vi "Idle Reference Image Window.vi"() -> ()   [LabVIEW 2017]
uses:
  Typedefs/Channel Selector.ctl
  Queue/Message Queue/Typedefs/Message Cluster.ctl
  SubVIs/Typedefs/Live window-ctrl refs.ctl
  Typedefs/Image display ref.ctl
  Typedefs/Save-Load enum.ctl
  <vilib>/Utility/miscctls.llb/LVPointTypeDef.ctl
  Typedefs/Read Write Enum.ctl
  Typedefs/Channel control synergistic behaviour enum.ctl
  Typedefs/Top level VI states.ctl
  Globals/gl_Windows Ctrl refs.vi
  Global Variables/General Globals.vi
  Global Variables/gl_UI Ctrl Refs.vi
panel:
  in  "UI queue ref control":refnum<queue>
  in  "Stop":bool
  in  "Show REF Image Right":bool caption="Show REF Image"
  in  "Show REF Image Left":bool caption="Show REF Image"
  in  "Base Path":path
  out "Frame rate (Hz)":dbl format="Acquisition frame rate: %.1f fps"
  in  "Sim multiplier":dbl(knob) scale=0.1..10.0
  out "Loop":i32
  out "Reset buffer":bool
  out "Refresh rate (Hz)":i32 format="Graph refresh rate: %.0f fps"
  in  "Right image intensity":cluster{i16, i16}(slide)={0, 804} scale=0.0..4095.0
  in  "Right Image Palette":enum16{"Gray", "Red", "Green"}(ring) caption="Palette"
  in  "Right Channel":T1=enum."Green Channel"
  in  "Left image intensity":cluster{i16, i16}(slide)={0, 871} scale=0.0..4095.0
  in  "Left Image Palette":enum16{"Gray", "Red", "Green"}(ring) caption="Palette"
  in  "Left Channel":T1
  in  "Y-scaling sensitivity":i32(slide)=32 scale=100.0..1.0
  in  "Sim":bool
  in  "AutoY once":bool
  in  "Selected Waveform":enum16{"Left graph", "Right graph"}(ring) caption="Displayed data"
  in  "Adaptive scaling is on":bool
  out "multiple tone information":T2(array[cluster])=[{"detected frequency"=59.40457132494078, "detected amplitude"=677.5224683183739, "detected phase (deg)"=-6.85916777032908}, {"detected frequency"=10023.302847711435, "detected amplitude"=302.0949374874943, "detected phase (deg)"=265.4481634375171}, {"detected frequency"=20019.602268100927, "detected amplitude"=136.99007273675608, "detected phase (deg)"=123.98051462950585}, {"detected frequency"=30006.01918128676, "detected amplitude"=20.477000538882503, "detected phase (deg)"=-16.173557072223005}] {"detected phase (deg)" format="%_6g"; "detected amplitude" format="%_6p"; "detected frequency" format="%_6p"}
  out "Right Image":T3(plugin-control)
  in  "Snapshot":bool
  out "Left Image":T3(plugin-control)
  out "Data graph":waveform(dbl)(graph)
  # "DO NOT DELETE THIS CONTROL. IT IS REFERENCED."
  # "Low                                   High"
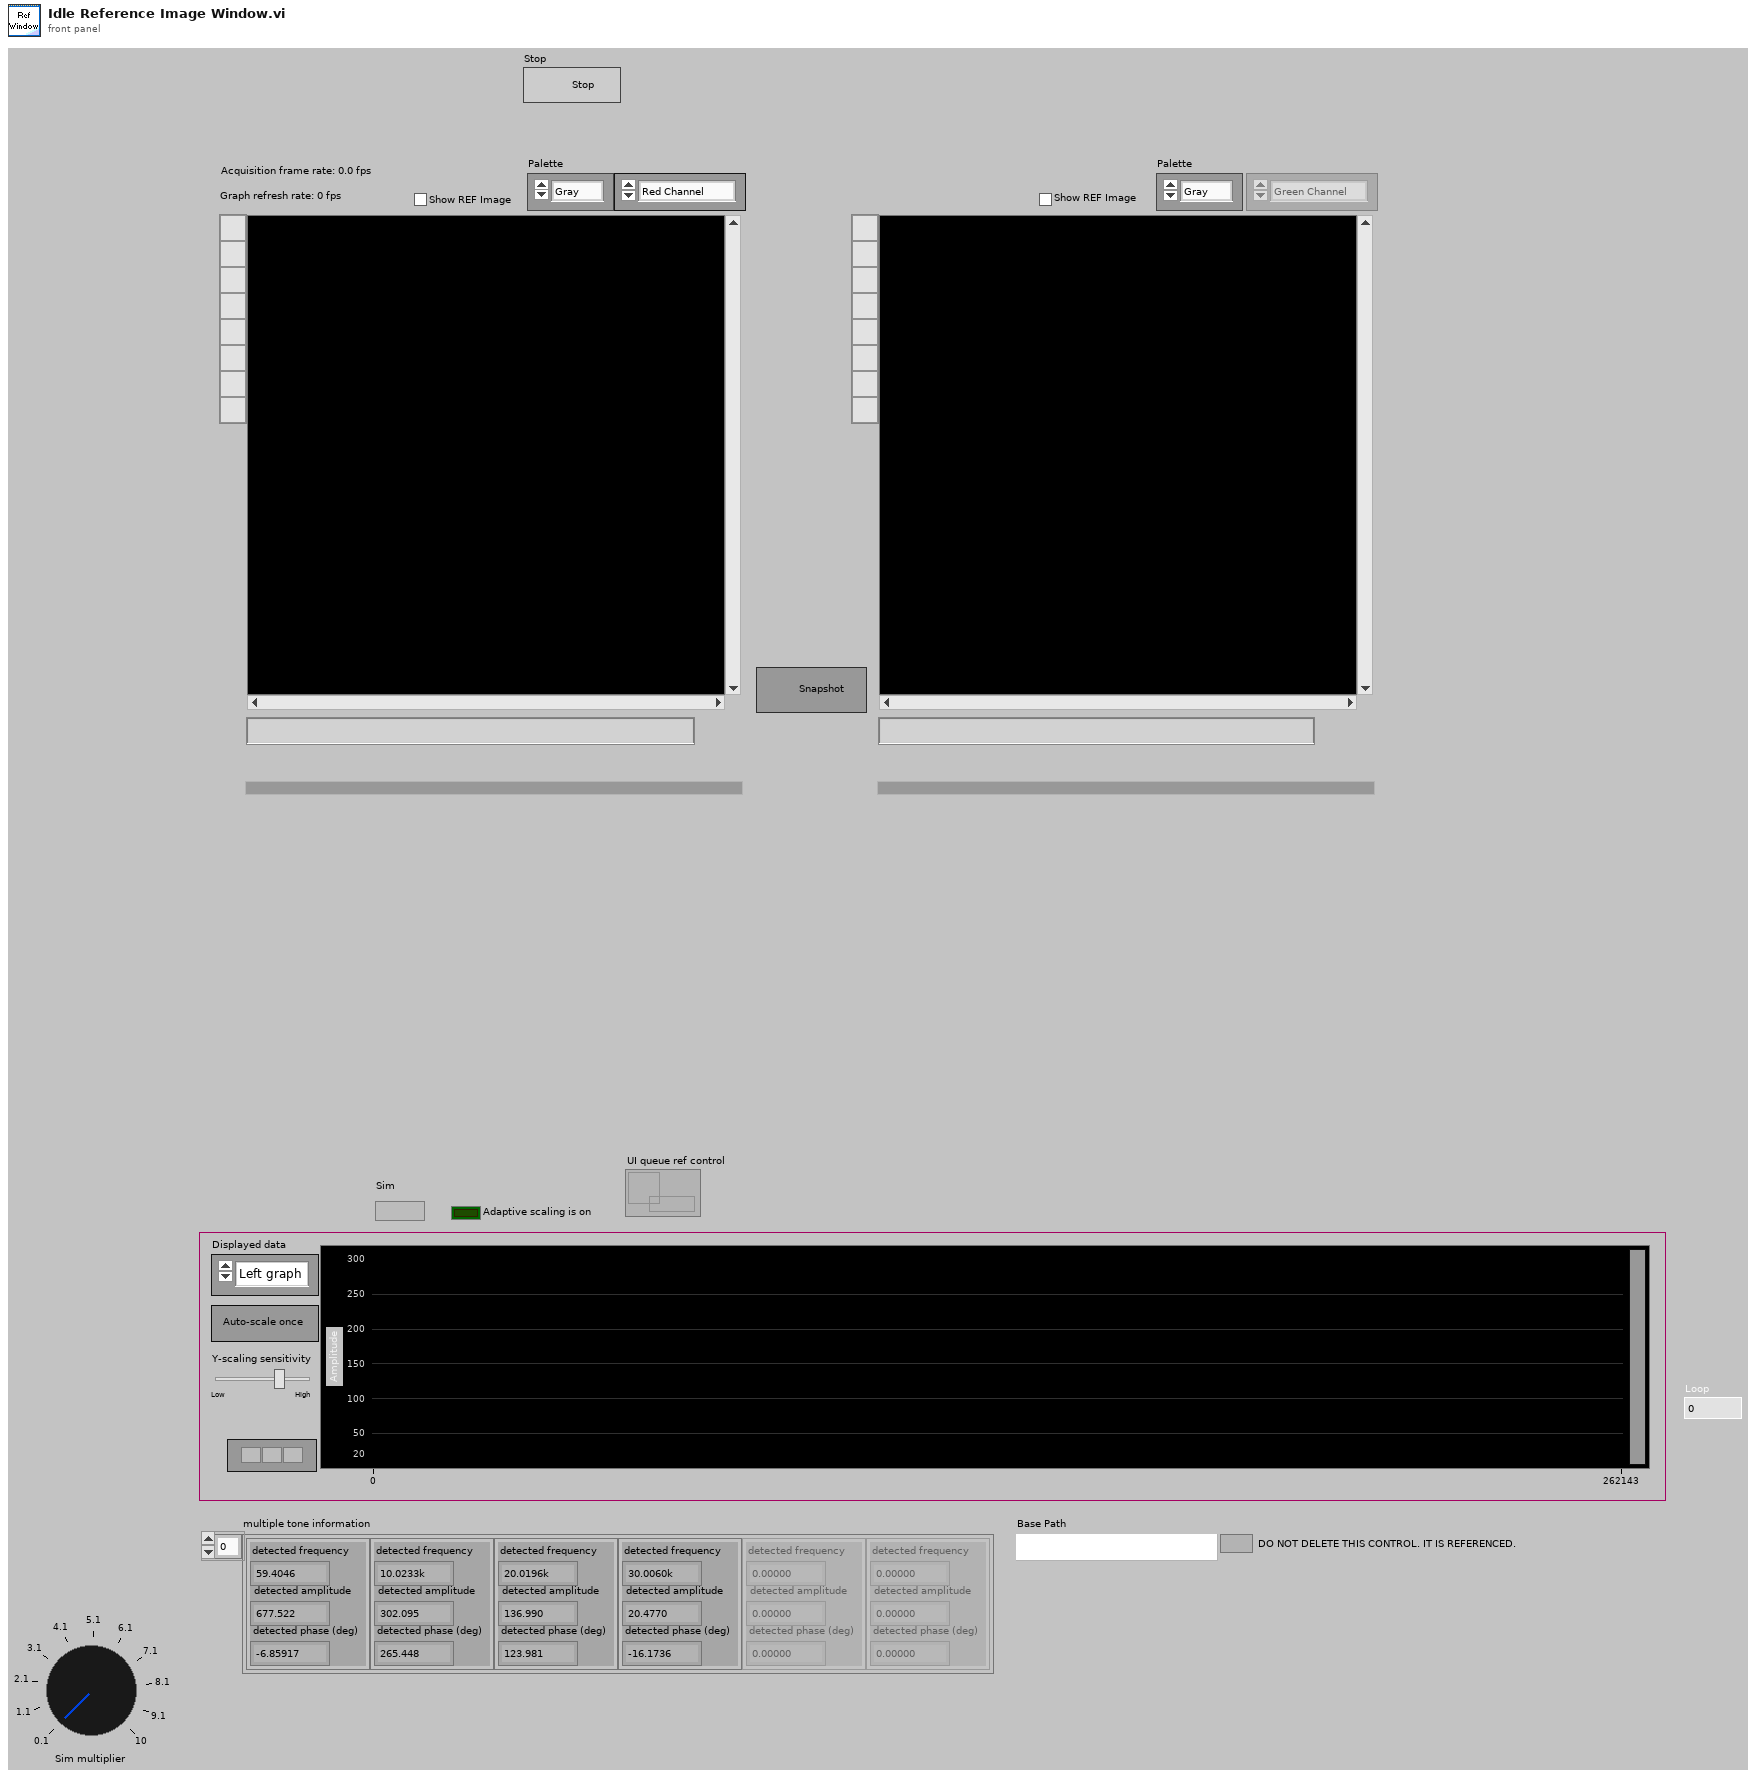
[diagram p1: front panel]
types:
  T1 = typedef "Channel Selector.ctl" = enum16{"Red Channel", "Green Channel", "Blended"}
  T2 = cluster{"detected frequency":dbl, "detected amplitude":dbl, "detected phase (deg)":dbl}[]
  T3 = typedef "IMAQ Image.ctl" = refnum<image>
  T4 = typedef "Live window-ctrl refs.ctl" = cluster{"This VI":refnum<vi>, "Pane":refnum<vi>, "Show REF Image Left":refnum<vi>, "Show REF Image Right":refnum<vi>, "Snapshot":refnum<vi>, "Left Image Palette":refnum<vi>, "Right Image Palette":refnum<vi>, "Left Channel":refnum<vi>, "Right Channel":refnum<vi>, "Left image intensity":refnum<vi>, "Right image intensity":refnum<vi>, "Left Image Display":T5, "Right Image Display":T5, "Refresh rate ind (Hz)":refnum<vi>, "Acq rate ind (Hz)":refnum<vi>, "Stop (ind)":refnum<vi>}
  T5 = typedef "Image display ref.ctl" = refnum<vi>
  T6 = typedef "Save-Load enum.ctl" = enum16{"Save to file", "Load from file", "Compare from file"}
  T7 = typedef "Read Write Enum.ctl" = enum16{"Read", "Write"}
  T8 = cluster{"Conversion Method":u32, "Minimum Value":i32, "Maximum Value":i32, "Number Of Shifts":i32}
  T9 = typedef "LVPointTypeDef.ctl" = cluster{"Horizontal":i16, "Vertical":i16}
  T10 = typedef "UI ctrl refs cluster.ctl" = cluster{"Top level VI path":path, "Top level VI ref":refnum<vi>, "User menu ref":refnum<k9>, "Sub Panel control":refnum<vi>, "Imaging Param Tab":refnum<vi>, "Occurrence-Start drivers":refnum<k4>, "Occurrence-Speed logging initialised":refnum<k4>, "Occurrence-XYZ stage initialised":refnum<k4>, "Exit button":refnum<vi>, "Status ind":refnum<vi>, "Set as origin":refnum<vi>, "Speed Logging":refnum<vi>, "Time Lapse":refnum<vi>, "Live Imaging":refnum<vi>, "AOL Z Stack":refnum<vi>, "Motor Z Stack":refnum<vi>, "Funct Acq button":refnum<vi>, "Hard Shutter":refnum<vi>, "Virtual Shutter":refnum<vi>, "Laser Power":refnum<vi>, "AOL Mode":refnum<vi>, "Frame Size":refnum<vi>, "Field of View":refnum<vi>, "Dwell Time":refnum<vi>, "Zoom":refnum<vi>, "AOL Z":refnum<vi>, "Objective":refnum<vi>, "Axis":refnum<vi>, "Paths & Names":refnum<vi>, "Experiment folder path (ind.)":refnum<vi>, "Last State (Ind.)":refnum<vi>, "Averages":refnum<vi>, "Angle (degrees)":refnum<vi>, "X centre":refnum<vi>, "Y centre":refnum<vi>, "Plane Mode":refnum<vi>, "# Planes":refnum<vi>, "Z Start":refnum<vi>, "Z Stop":refnum<vi>, "Z Step":refnum<vi>, "PMT 1":refnum<vi>, "PMT 2":refnum<vi>, "Stage XYZ Position":refnum<vi>, "Pockels@Z Start":refnum<vi>, "Pockels@Z Stop":refnum<vi>, "Obtain Z Start":refnum<vi>, "Obtain Z Stop":refnum<vi>, "Live stim.trig.period":refnum<vi>, "Live stim.trig.enable":refnum<vi>, "Movement Correction":refnum<vi>, "Load Reference Image":refnum<vi>, "XY Stage Move":refnum<vi>, "MovCor Cluster":refnum<vi>, "RefDAQParam":refnum<vi>, "Funct. Acq. Pockels Modulation":refnum<vi>, "Ref Laser Power":refnum<vi>, "Enable Video Recording":refnum<vi>, "Video Record-Live Imaging":refnum<vi>, "Video Record-Funct acq":refnum<vi>, "Reference Source":refnum<vi>, "AOL Z-stack Chirps Ready (ind)":refnum<vi>, "Target time between mov.cor. ref triggers (ms)":refnum<vi>, "Funct. Acq. Ref frame save":refnum<vi>, "Tracking button":refnum<vi>, "Show ref plots window":refnum<vi>, "Center freq ind (nm)":refnum<vi>, "Pickup mode (ind)":refnum<vi>, "Logging queue (ind)":refnum<vi>, "Back aperture power (ind.)":refnum<vi>, "Power after objective (ind.)":refnum<vi>, "Switch user":refnum<vi>, "Ls1 Conn. Status":refnum<vi>, "Ls1Tuning Status":refnum<vi>, "Ls1 Faults":refnum<vi>, "Ls1 Connection":refnum<vi>, "Ls1 Mode":refnum<vi>, "Ls1 POWER [mW]":refnum<vi>, "Ls1Shutter":refnum<vi>, "Ls1 Wavelength":refnum<vi>, "Ls1 Note":refnum<vi>, "Ls1 Confirm Wav":refnum<vi>, "Ls1 PreChrp Prism1":refnum<vi>, "Ls1 PreChrp Prism2":refnum<vi>, "Ls1 wav top Ind":refnum<vi>, "Ls1 power top Ind":refnum<vi>, "Ls1 Pump peak Hold":refnum<vi>, "Ls1 Status Ind":refnum<vi>, "Ls1 wav cancel":refnum<vi>, "Experiment Type":refnum<vi>, "Biology Information":refnum<vi>}
  T11 = typedef "Live graph data queue ref.ctl" = refnum<queue>
  T12 = typedef "Channel control synergistic behaviour enum.ctl" = enum16{"Left disabled-Right enabled", "Left enabled-Right disabled", "Both enabled"}
  T13 = cluster{"Caption-Right button":string, "Caption-Left button":string, "Message to display":string, "Delay before close":u32, "Window Colour":u32, "Cancel button disabled?":enum8{"Enabled", "Disabled", "Disabled and Grayed Out"}}
  T14 = typedef "Top level VI states.ctl" = enum16{"None", "Initialise UI", "<STACK PROTOCOL STATES>", "AOL Zstack-START", "AOL Zstack-STOP", "Motor Zstack-START", "Motor Zstack-STOP", "<ACQUISITION PROTOCOL STATES> ", "Functional Acquisition-START", "Functional Acquisition-STOP", "Single Plane Acquisition-START", "Single Plane Acquisition-STOP", "Volume Acquisition-START", "Volume Acquisition-STOP", "<LIVE IMAGING PROTOCOL STATES>", "Live Imaging-START", "Live Imaging-STOP", "Live Plane Imaging-START", "Live Plane Imaging-STOP", "Live Volume Imaging-START", "Live Volume Imaging-STOP", "<MOVEMENT CORRECTION PROTOCOL STATES>", "EXIT"}
  T15 = typedef "Live imaging queue element.ctl" = cluster{"Red channel":T3, "Green channel":T3, "Ref Red channel":T3, "Ref Green channel":T3, "Mov cor":bool}
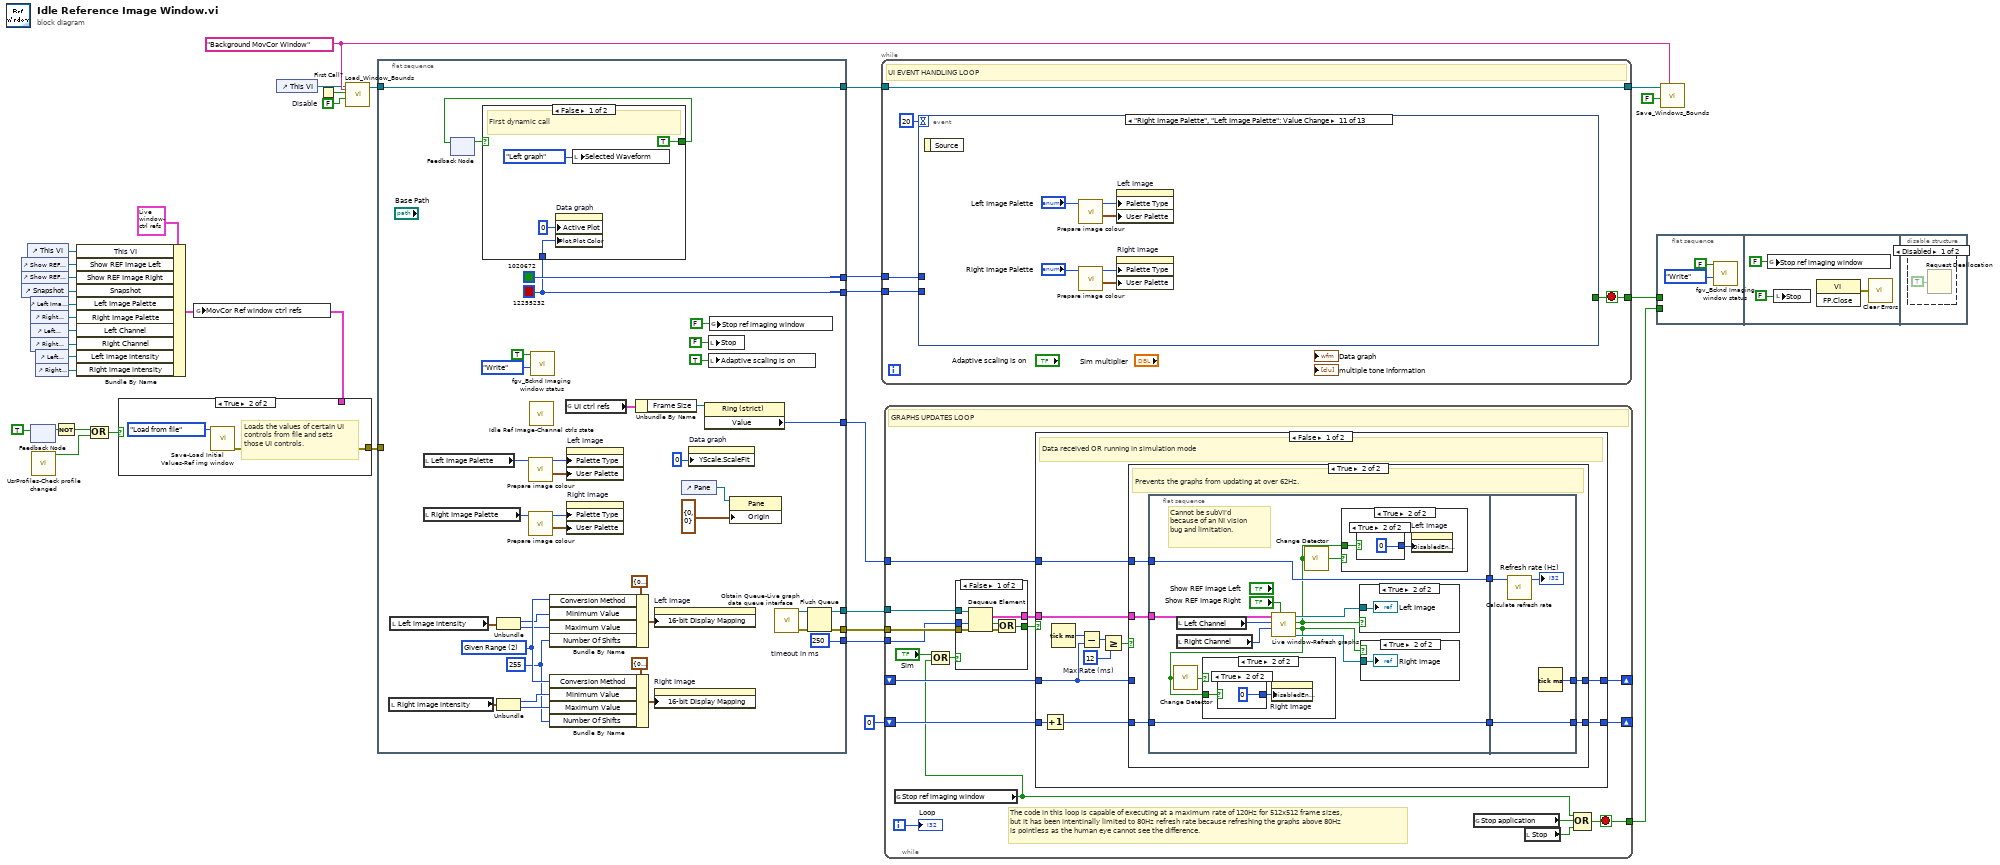
[diagram p0: block diagram]
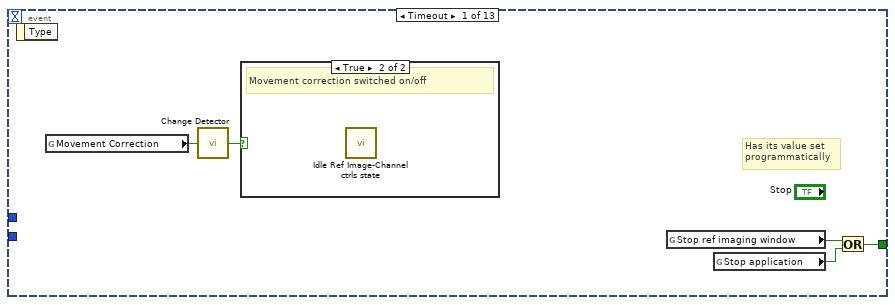
[diagram p5: hidden frame]
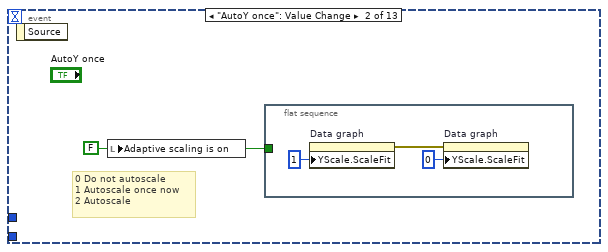
[diagram p7: hidden frame]
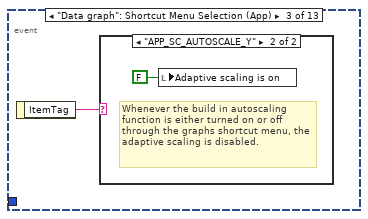
[diagram p8: hidden frame]
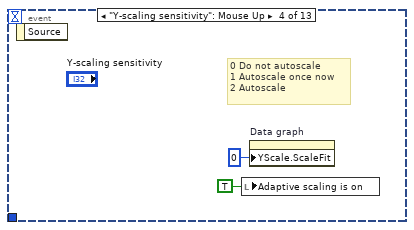
[diagram p10: hidden frame]
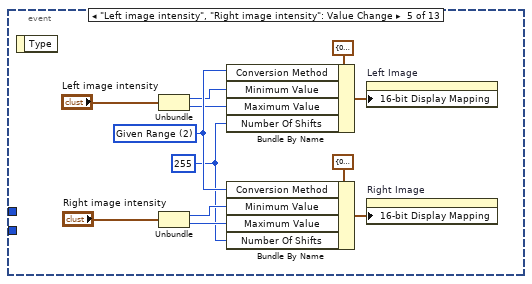
[diagram p11: hidden frame]
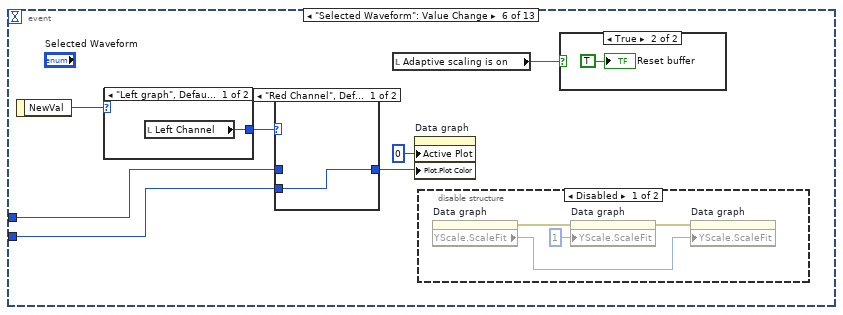
[diagram p12: hidden frame]
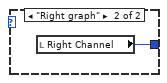
[diagram p16: hidden frame]
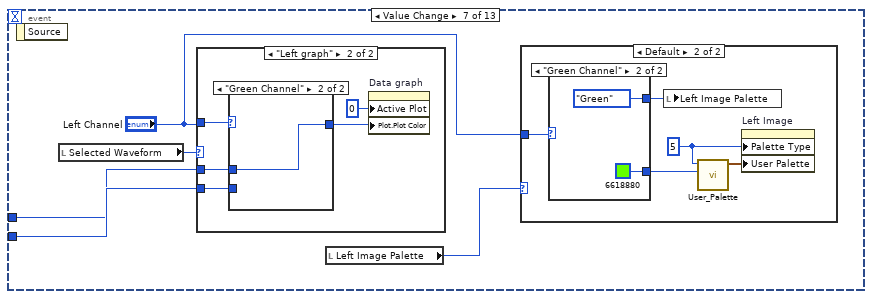
[diagram p17: hidden frame]
diagram:
  w31 = FALSE  # Disable
  w30 = "Background MovCor Window" ("Window Name (i.e. Key)")
  n1 = control-ref of="Show REF Image Left"() -> (w15:refnum<vi>)
  n2 = control-ref of="Show REF Image Right"() -> (w16:refnum<vi>)
  n3 = control-ref of="Snapshot"() -> (w17:refnum<vi>)
  n4 = control-ref of="This VI"() -> (w14:refnum<vi>)
  n5 = control-ref of="Left Image Palette"() -> (w11:refnum<vi>)
  n6 = control-ref of="Right Image Palette"() -> (w10:refnum<vi>)
  n7 = control-ref of="Left Channel"() -> (w9:refnum<vi>)
  n8 = control-ref of="Right Channel"() -> (w8:refnum<vi>)
  n9 = feedback #1() -> (w5:bool)  [unwired: 1 in]
  n10 = feedback-in #1(TRUE) -> ()
  n11 = call "UsrProfiles-Check profile changed.vi"() -> ("Profile changed"=w1:bool)  [unwired: 10 in, 1 out]
  n12 = control-ref of="Left image intensity"() -> (w7:refnum<vi>)
  n13 = control-ref of="Right image intensity"() -> (w6:refnum<vi>)
  n14 = Not(x=w5) -> (.not. x?=w3:bool)
  n15 = Bundle By Name(cluster=T4 {"This VI"=refnum, "Pane"=refnum, "Show REF Image Left"=refnum, "Show REF Image Right"=refnum, "Snapshot"=refnum, "Left Image Palette"=refnum, "Right Image Palette"=refnum, "Left Channel"=refnum, "Right Channel"=refnum, "Left image intensity"=refnum, "Right image intensity"=refnum, "Left Image Display"=refnum, "Right Image Display"=refnum, "Refresh rate ind (Hz)"=refnum, "Acq rate ind (Hz)"=refnum, "Stop (ind)"=refnum} ("Live imaging window ctrl refs"), "This VI"=w14, "Show REF Image Left"=w15, "Show REF Image Right"=w16, "Snapshot"=w17, "Left Image Palette"=w11, "Right Image Palette"=w10, "Left Channel"=w9, "Right Channel"=w8, "Left image intensity"=w7, "Right image intensity"=w6) -> (w12:T4)
  n16 = Compound Arithmetic op=OR(w3, w1) -> (w2:bool)
  n17 = case shown="True" w2 {
    tunnel: [_ w36] -> w18
    tunnel: w12 -> [_ _]
    frame False {
    }
    frame True {
      # "Loads the values of certain UI controls from file and sets those UI controls."
      n18 = call "Save-Load Initial Values-Ref img window.vi"("Function"=Save-Load_enum."Load from file") -> ("error out"=w36:errorcluster)  [unwired: 10 in]
    }
  }
  n19 = global write "gl_Windows Ctrl refs.vi" "MovCor Ref window ctrl refs"(w12) -> ()
  n20 = control-ref of="This VI"() -> (w24:refnum<vi>)
  n21 = First Call?() -> (First Call?: T/F=w32:bool)
  n22 = call "Load_Window_Bounds.vi"("Window Name (i.e. Key)"=w30, "Disable"=w31, "First Call"=w32, "Window VI's Ref"=w24) -> ("reference out"=w19:refnum<vi>)  [unwired: 4 in, 3 out]
  n23 = flat-sequence {
    tunnel: [u32 1020672 ("Green")] -> w35
    tunnel: [w75] -> w34
    tunnel: [w72] -> w33
    tunnel: w19 -> [w44]
    tunnel: [w44] -> w23
    tunnel: [w41] -> w22
    tunnel: [w40] -> w21
    tunnel: [w42] -> w20
    tunnel: w18 -> [_]
    frame #0 {
      w42 = 250  # timeout in ms
      w57 = 255 ("Number Of Shifts")
      w65 = u32 2 items=["Full Dynamic", "Downshift", "Given Range", "90% Dynamic", "Given Percent Range"] ("16-bit Display Mapping:Conversion Method")
      w75 = u32 12255232 ("Red")
      n24 = local read "Right image intensity"() -> (w67:cluster{i16, i16})
      n25 = local read "Left image intensity"() -> (w66:cluster{i16, i16})
      n26 = local read "Left Image Palette"() -> (w49:enum16{"Gray", "Red", "Green"})
      n27 = local read "Right Image Palette"() -> (w48:enum16{"Gray", "Red", "Green"})
      n28 = feedback #2() -> (w74:bool)  [unwired: 1 in]
      n29 = case shown="False" w74 {
        selector: w74 -> [_ w81]
        tunnel: w75 -> [w78 _]
        tunnel: [TRUE w81] -> w73
        frame False {
          # "First dynamic call"
          n30 = property on="Data graph" class="MixedGraph (strict)"("Active Plot"=u32 0, "Plot.Plot Color"=w78) -> ()  [unwired: 2 in, 2 out]
          n31 = local write "Selected Waveform"(enum16{"Left graph", "Right graph"}."Left graph" ("Selected Waveform")) -> ()
        }
        frame True {
          # "Consecutive calls"
        }
      }
      n32 = feedback-in #2(w73) -> ()
      n33 = Unbundle(w66) -> (w61:i16, w62:i16)
      n34 = Unbundle(w67) -> (w64:i16, w63:i16)
      n35 = call "Prepare image colour.vi"("Left Image Palette"=w49) -> ("Color Palette"=w52:cluster{"Red":u8, "Green":u8, "Blue":u8}[], "Palette Type"=w50:u32)  [unwired: 8 in, 1 out]
      n36 = call "Prepare image colour.vi"("Left Image Palette"=w48) -> ("Color Palette"=w53:cluster{"Red":u8, "Green":u8, "Blue":u8}[], "Palette Type"=w51:u32)  [unwired: 8 in, 1 out]
      n37 = call "Idle Ref Image-Channel ctrls state.vi"() -> ()  [unwired: 12 in]
      n38 = call "fgv_Bcknd Imaging window status.vi"("Function"=Read_Write_Enum."Write", "Background MovCor window is open"=TRUE) -> ()  [unwired: 8 in, 2 out]
      n39 = Bundle By Name(cluster=T8 {"Conversion Method"=0, "Minimum Value"=0, "Maximum Value"=0, "Number Of Shifts"=0} ("16-bit Display Mapping:All Elements"), "Conversion Method"=w65, "Minimum Value"=w61, "Maximum Value"=w62, "Number Of Shifts"=w57) -> (w59:T8)
      n40 = Bundle By Name(cluster=T8 {"Conversion Method"=0, "Minimum Value"=0, "Maximum Value"=0, "Number Of Shifts"=0} ("16-bit Display Mapping:All Elements"), "Conversion Method"=w65, "Minimum Value"=w64, "Maximum Value"=w63, "Number Of Shifts"=w57) -> (w58:T8)
      n41 = global read "gl_UI Ctrl Refs.vi" "UI ctrl refs"() -> (w54:T10)
      n42 = property on="Left Image" class="ImageControl"("Palette Type"=w50, "User Palette"=w52) -> ()  [unwired: 2 in, 2 out]
      n43 = property on="Right Image" class="ImageControl"("Palette Type"=w51, "User Palette"=w53) -> ()  [unwired: 2 in, 2 out]
      n44 = Unbundle By Name(w54) -> ("Frame Size"=w55:refnum<vi>)
      n45 = property on="Left Image" class="ImageControl"("16-bit Display Mapping"=w59) -> ()  [unwired: 2 in, 2 out]
      n46 = property on="Right Image" class="ImageControl"("16-bit Display Mapping"=w58) -> ()  [unwired: 2 in, 2 out]
      n47 = control-ref of="Pane"() -> (w70:refnum<vi>)
      n48 = property on="Data graph" class="MixedGraph (strict)"("YScale.ScaleFit"=u8 0 ("Y Scale.Scale Fit")) -> ()  [unwired: 2 in, 2 out]
      n49 = property class="Ring (strict)"(reference=w55) -> ("Value"=w72:u16)  [unwired: 1 in, 2 out]
      n50 = local write "Stop"(FALSE ("Stop")) -> ()
      n51 = local write "Adaptive scaling is on"(TRUE ("Custom scaling on")) -> ()
      n52 = global write "General Globals.vi" "Stop ref imaging window"(FALSE ("Stop ref imaging window")) -> ()
      n53 = property class="Pane"(reference=w70, "Origin"=T9 {"Horizontal"=0, "Vertical"=0}) -> ()  [unwired: 1 in, 2 out]
      n54 = call "Obtain Queue-Live graph data queue interface.vi"() -> ("error out"=w39:errorcluster, "Live graphs queue"=w43:T11)  [unwired: 10 in]
      n55 = Flush Queue(queue=w43, error in (no error)=w39) -> (queue out=w41:T11, error out=w40:errorcluster)  [unwired: 1 out]
    }
  }
  n56 = while {
    tunnel: [w85] -> w26
    tunnel: w34 -> [w84]
    tunnel: w35 -> [w83]
    tunnel: [w82] -> w28
    tunnel: w23 -> [w82]
    stop <- w85 stop-if-true
    # "UI EVENT HANDLING LOOP"
    n57 = event shown="[10] \"Right Image Palette\", \"Left Image Palette\": Value Change" {
      selector: _ -> [_ _ _ _ _ _ _ _ _ _ _ _ _]
      dyn-events: _ -> [_ _ _ _ _ _ _ _ _ _ _ _ _]
      timeout: 20 -> [_ _ _ _ _ _ _ _ _ _ _ _ _]
      tunnel: [w91 _ _ _ _ _ _ _ _ _ _ _ w188] -> w85
      tunnel: w84 -> [_ _ _ _ _ w113 w131 _ _ w160 _ _ _]
      tunnel: w83 -> [_ _ _ _ _ w114 w130 _ _ w161 _ _ _]
      event Timeout {
        # "Has its value set \nprogrammatically"
        n58 = event-data() -> ()  [unwired: 1 in, 1 out]
        n59 = global read "General Globals.vi" "Movement Correction"() -> (w87:bool)
        n60 = call <userlib>:"Change Detector.vi"("Value"=w87) -> ("Changed?"=w88:bool)
        n61 = case shown="True" w88 {
          frame False {
            # "Idle"
          }
          frame True {
            # "Movement correction switched on/off"
            n62 = call "Idle Ref Image-Channel ctrls state.vi"() -> ()  [unwired: 12 in]
          }
        }
        n63 = global read "General Globals.vi" "Stop ref imaging window"() -> (w89:bool)
        n64 = global read "General Globals.vi" "Stop application"() -> (w90:bool)
        n65 = Or(x=w89, y=w90) -> (x .or. y?=w91:bool)
      }
      event "AutoY once": Value Change {
        w92 = FALSE ("Custom scaling on")
        # "0 Do not autoscale \n1 Autoscale once now \n2 Autoscale"
        n66 = event-data() -> ()  [unwired: 1 in, 1 out]
        n67 = local write "Adaptive scaling is on"(w92) -> ()
        n68 = flat-sequence {
          tunnel: w92 -> [_]
          frame #0 {
            n69 = property on="Data graph" class="MixedGraph (strict)"("YScale.ScaleFit"=u8 1 ("Y Scale.Scale Fit")) -> (error out=w93:errorcluster)  [unwired: 2 in, 1 out]
            n70 = property on="Data graph" class="MixedGraph (strict)"(error in=w93, "YScale.ScaleFit"=u8 0 ("Y Scale.Scale Fit")) -> ()  [unwired: 1 in, 2 out]
          }
        }
      }
      event "Data graph": Shortcut Menu Selection (App) {
        n71 = event-data() -> ("ItemTag"=w96:string)  [unwired: 1 in]
        n72 = case shown="\"APP_SC_AUTOSCALE_Y\"" w96 {
          frame Default {
          }
          frame "APP_SC_AUTOSCALE_Y" {
            # "Whenever the build in autoscaling function is either turned on or off through the graphs shortcut menu, the adaptive scaling is disabled."
            n73 = local write "Adaptive scaling is on"(FALSE ("Custom scaling on")) -> ()
          }
        }
      }
      event "Y-scaling sensitivity": Mouse Up {
        # "0 Do not autoscale \n1 Autoscale once now \n2 Autoscale"
        n74 = event-data() -> ()  [unwired: 1 in, 1 out]
        n75 = local write "Adaptive scaling is on"(TRUE ("Custom scaling on")) -> ()
        n76 = property on="Data graph" class="MixedGraph (strict)"("YScale.ScaleFit"=u8 0 ("Y Scale.Scale Fit")) -> ()  [unwired: 2 in, 2 out]
      }
      event "Left image intensity", "Right image intensity": Value Change {
        w103 = 255 ("Number Of Shifts")
        w111 = u32 2 items=["Full Dynamic", "Downshift", "Given Range", "90% Dynamic", "Given Percent Range"] ("16-bit Display Mapping:Conversion Method")
        n77 = event-data() -> ()  [unwired: 1 in, 1 out]
        n78 = Unbundle("Left image intensity") -> (w107:i16, w108:i16)
        n79 = Unbundle("Right image intensity") -> (w110:i16, w109:i16)
        n80 = Bundle By Name(cluster=T8 {"Conversion Method"=0, "Minimum Value"=0, "Maximum Value"=0, "Number Of Shifts"=0} ("16-bit Display Mapping:All Elements"), "Conversion Method"=w111, "Minimum Value"=w107, "Maximum Value"=w108, "Number Of Shifts"=w103) -> (w105:T8)
        n81 = Bundle By Name(cluster=T8 {"Conversion Method"=0, "Minimum Value"=0, "Maximum Value"=0, "Number Of Shifts"=0} ("16-bit Display Mapping:All Elements"), "Conversion Method"=w111, "Minimum Value"=w110, "Maximum Value"=w109, "Number Of Shifts"=w103) -> (w104:T8)
        n82 = property on="Left Image" class="ImageControl"("16-bit Display Mapping"=w105) -> ()  [unwired: 2 in, 2 out]
        n83 = property on="Right Image" class="ImageControl"("16-bit Display Mapping"=w104) -> ()  [unwired: 2 in, 2 out]
      }
      event "Selected Waveform": Value Change {
        n84 = event-data() -> ("NewVal"=w118:enum16{"Left graph", "Right graph"})  [unwired: 1 in]
        n85 = case shown="\"Left graph\", Default" w118 {
          tunnel: [w126 w127] -> w115
          frame "Left graph", Default {
            n86 = local read "Left Channel"() -> (w126:T1)
          }
          frame "Right graph" {
            n87 = local read "Right Channel"() -> (w127:T1)
          }
        }
        n88 = case shown="\"Red Channel\", Default" w115 {
          tunnel: [w124 w125] -> w117
          tunnel: w114 -> [_ w125]
          tunnel: w113 -> [w124 _]
          frame "Red Channel", Default {
          }
          frame "Green Channel" {
          }
        }
        n89 = local read "Adaptive scaling is on"() -> (w112:bool)
        n90 = property on="Data graph" class="MixedGraph (strict)"("Active Plot"=u32 0, "Plot.Plot Color"=w117) -> ()  [unwired: 2 in, 2 out]
        n91 = disable-structure shown="Disabled" {
          frame Disabled {
            n92 = property on="Data graph" class="MixedGraph (strict)"() -> (error out=w121:errorcluster, "YScale.ScaleFit"=w120:u8)  [unwired: 2 in, 1 out]
            n93 = property on="Data graph" class="MixedGraph (strict)"(error in=w121, "YScale.ScaleFit"=u8 1 ("Y Scale.Scale Fit")) -> (error out=w122:errorcluster)  [unwired: 1 in, 1 out]
            n94 = property on="Data graph" class="MixedGraph (strict)"(error in=w122, "YScale.ScaleFit"=w120) -> ()  [unwired: 1 in, 2 out]
          }
          frame Enabled {
          }
        }
        n95 = case shown="True" w112 {
          frame False {
          }
          frame True {
            "Reset buffer" <- TRUE
          }
        }
      }
      event Value Change {
        n96 = event-data() -> ()  [unwired: 1 in, 1 out]
        n97 = local read "Selected Waveform"() -> (w129:enum16{"Left graph", "Right graph"})
        n98 = case shown="\"Left graph\"" w129 {
          tunnel: "Left Channel" -> [_ w137]
          tunnel: w131 -> [_ w134]
          tunnel: w130 -> [_ w133]
          frame Default {
          }
          frame "Left graph" {
            n99 = case shown="\"Green Channel\"" w137 {
              tunnel: [w138 w139] -> w136
              tunnel: w133 -> [_ w139]
              tunnel: w134 -> [w138 _]
              frame "Red Channel", Default {
              }
              frame "Green Channel" {
              }
            }
            n100 = property on="Data graph" class="MixedGraph (strict)"("Active Plot"=u32 0, "Plot.Plot Color"=w136) -> ()  [unwired: 2 in, 2 out]
          }
        }
        n101 = local read "Left Image Palette"() -> (w128:enum16{"Gray", "Red", "Green"})
        n102 = case shown="Default" w128 {
          tunnel: "Left Channel" -> [_ w143]
          frame "Gray" {
          }
          frame Default {
            w140 = u32 5 ("t")
            n103 = case shown="\"Green Channel\"" w143 {
              tunnel: [enum16{"Gray", "Red", "Green"}."Red" ("Left Image Palette") enum16{"Gray", "Red", "Green"}."Green" ("Left Image Palette")] -> w142
              tunnel: [u32 16711680 ("Color") u32 6618880 ("Color")] -> w141
              frame "Red Channel", Default {
              }
              frame "Green Channel" {
              }
            }
            n104 = local write "Left Image Palette"(w142) -> ()
            n105 = call "User_Palette.vi"("Color"=w141, "Palette Number (gray)"=w140) -> ("Color Palette"=w144:cluster{"Red":u8, "Green":u8, "Blue":u8}[])  [unwired: 9 in]
            n106 = property on="Left Image" class="ImageControl"("Palette Type"=w140, "User Palette"=w144) -> ()  [unwired: 2 in, 2 out]
          }
        }
      }
      event "Show REF Image Left": Value Change {
        n107 = event-data() -> ("OldVal"=w150:bool)  [unwired: 1 in]
        n108 = local write "Show REF Image Right"(w150) -> ()
        n109 = Select(t=Channel_control_synergistic_behaviour_enum."Left disabled-Right enabled" ("Behaviour"), s=w150, f=Channel_control_synergistic_behaviour_enum."Left enabled-Right disabled" ("Behaviour")) -> (s? t:f=w149:T12)
        n110 = call "Channel ctrl disabled synergy-Bgnd MovCor.vi"("Behaviour"=w149) -> ()  [unwired: 10 in, 1 out]
      }
      event "Show REF Image Right": Value Change {
        n111 = event-data() -> ("OldVal"=w155:bool)  [unwired: 1 in]
        n112 = local write "Show REF Image Left"(w155) -> ()
        n113 = Select(t=Channel_control_synergistic_behaviour_enum."Left enabled-Right disabled" ("Behaviour"), s=w155, f=Channel_control_synergistic_behaviour_enum."Left disabled-Right enabled" ("Behaviour")) -> (s? t:f=w156:T12)
        n114 = call "Channel ctrl disabled synergy-Bgnd MovCor.vi"("Behaviour"=w156) -> ()  [unwired: 10 in, 1 out]
      }
      event Value Change {
        n115 = event-data() -> ()  [unwired: 1 in, 1 out]
        n116 = local read "Selected Waveform"() -> (w159:enum16{"Left graph", "Right graph"})
        n117 = case shown="\"Right graph\"" w159 {
          tunnel: "Right Channel" -> [_ w166]
          tunnel: w161 -> [_ w163]
          tunnel: w160 -> [_ w162]
          frame Default {
          }
          frame "Right graph" {
            n118 = case shown="\"Red Channel\", Default" w166 {
              tunnel: [w167 w168] -> w165
              tunnel: w163 -> [_ w168]
              tunnel: w162 -> [w167 _]
              frame "Red Channel", Default {
              }
              frame "Green Channel" {
              }
            }
            n119 = property on="Data graph" class="MixedGraph (strict)"("Active Plot"=u32 0, "Plot.Plot Color"=w165) -> ()  [unwired: 2 in, 2 out]
          }
        }
        n120 = local read "Right Image Palette"() -> (w158:enum16{"Gray", "Red", "Green"})
        n121 = case shown="Default" w158 {
          tunnel: "Right Channel" -> [_ w172]
          frame "Gray" {
          }
          frame Default {
            w170 = u32 5 ("t")
            n122 = case shown="\"Green Channel\"" w172 {
              tunnel: [enum16{"Gray", "Red", "Green"}."Red" ("Left Image Palette") enum16{"Gray", "Red", "Green"}."Green" ("Left Image Palette")] -> w169
              tunnel: [u32 16711680 ("Color") u32 6618880 ("Color")] -> w171
              frame "Red Channel", Default {
              }
              frame "Green Channel" {
              }
            }
            n123 = local write "Right Image Palette"(w169) -> ()
            n124 = call "User_Palette.vi"("Color"=w171, "Palette Number (gray)"=w170) -> ("Color Palette"=w173:cluster{"Red":u8, "Green":u8, "Blue":u8}[])  [unwired: 9 in]
            n125 = property on="Right Image" class="ImageControl"("Palette Type"=w170, "User Palette"=w173) -> ()  [unwired: 2 in, 2 out]
          }
        }
      }
      event "Right Image Palette", "Left Image Palette": Value Change {
        n126 = event-data() -> ()  [unwired: 1 in, 1 out]
        n127 = call "Prepare image colour.vi"("Left Image Palette"="Left Image Palette") -> ("Color Palette"=w180:cluster{"Red":u8, "Green":u8, "Blue":u8}[], "Palette Type"=w183:u32)  [unwired: 8 in, 1 out]
        n128 = call "Prepare image colour.vi"("Left Image Palette"="Right Image Palette") -> ("Color Palette"=w179:cluster{"Red":u8, "Green":u8, "Blue":u8}[], "Palette Type"=w181:u32)  [unwired: 8 in, 1 out]
        n129 = property on="Left Image" class="ImageControl"("Palette Type"=w183, "User Palette"=w180) -> ()  [unwired: 2 in, 2 out]
        n130 = property on="Right Image" class="ImageControl"("Palette Type"=w181, "User Palette"=w179) -> ()  [unwired: 2 in, 2 out]
      }
      event "Snapshot": Value Change {
        # "The button's behaviour has been set to \"Switch when pressed\" on purpose to eliminate a UI redraw issue."
        n131 = event-data() -> ("NewVal"=w186:bool)  [unwired: 1 in]
        n132 = local read "Left Image"() -> (w187:T3)
        n133 = local read "Right Image"() -> (w185:T3)
        n134 = global read "gl_Windows Ctrl refs.vi" "MovCor Ref window ctrl refs"() -> (w184:T4)
        n135 = call "Live window-Snapshot handler.vi"("Window ctrl refs"=w184, "Right image"=w185, "Left image"=w187, "Snapshot:NewVal"=w186) -> ()  [unwired: 8 in]
      }
      event Panel Close? {
        n136 = event-data() -> ()  [unwired: 1 in, 4 out]
        n137 = flat-sequence {
          tunnel: [w196] -> w190
          tunnel: [w198] -> w188
          tunnel: w190 -> [w197]
          frame #0 {
            n138 = Bundle By Name(cluster=T13 {"Caption-Right button"="", "Caption-Left button"="", "Message to display"="", "Delay before close"=0, "Window Colour"=16448250, "Cancel button disabled?"=enum."Enabled"} ("Input cluster"), "Caption-Right button"="Close & Disable", "Caption-Left button"="Cancel", "Message to display"="If you close this window background movement correction will be disabled.") -> (w194:T13)
            n139 = call "Window-User dialogue.vi"("Input cluster"=w194) -> ("Left Button (Cancel)"=w196:bool)  [unwired: 10 in]
          }
          frame #1 {
            n140 = case shown="False" w197 {
              tunnel: [TRUE ("Stop") FALSE ("Stop")] -> w198
              frame False {
                w200 = FALSE  # Bcgnd movcor enabled?
                w201 = FALSE  # Also grey out?
                # "Disables the Bckgnd MovCor"
                # "Proceed"
                n141 = call "Request Background Movement Correction STOP.vi"("Next State"=Top_level_VI_states."None", "UI queue in"="UI queue ref control") -> ("error out"=w202:errorcluster)  [unwired: 8 in, 1 out]
                n142 = call "Set Background MovCor Global and Control.vi"("Also grey out?"=w201, "On/Off"=w200) -> ()  [unwired: 9 in, 1 out]
                n143 = call <vilib>:"Clear Errors.vi"("error in (no error)"=w202) -> ()  [unwired: 5 in, 2 out]
              }
              frame True {
                # "Cancelled"
              }
            }
          }
        }
        n144 = Not(x=w188) -> (.not. x?=w189:bool)
        n145 = local write "Stop"(w188) -> ()
        n146 = event-data("Discard?"=w189) -> ()  [unwired: 1 in, 1 out]
      }
    }
  }
  n147 = while {
    tunnel: w22 -> [w222]
    tunnel: w21 -> [w221]
    tunnel: w20 -> [w218]
    shift-right: [w216] -> _
    shift-left: 0 -> [w212]
    tunnel: w33 -> [w215]
    shift-right: [w214] -> _
    shift-left: _ -> [w213]
    tunnel: [w209] -> w25
    i -> [w217]
    stop <- w209 stop-if-true
    # "The code in this loop is capable of executing at a maximum rate of 120Hz for 512x512 frame sizes,\nbut it has been intentinally limited to 80Hz refresh rate because refreshing the graphs above 80Hz\nis pointless as the human eye cannot see the difference."
    # "GRAPHS UPDATES LOOP"
    n148 = global read "General Globals.vi" "Stop ref imaging window"() -> (w208:bool)
    n149 = Compound Arithmetic op=OR("Sim", w208) -> (w206:bool)
    n150 = case shown="False" w206 {
      tunnel: [w229 _] -> w220
      tunnel: w222 -> [w228 _]
      tunnel: w221 -> [w227 _]
      tunnel: w218 -> [w226 _]
      tunnel: [w224 FALSE ("timed out?")] -> w219
      frame False {
        n151 = Dequeue Element(queue=w228, timeout in ms (-1)=w226, error in (no error)=w227) -> (element=w229:T15, timed out?=w225:bool, error out=w223:errorcluster)  [unwired: 1 out]
        n152 = Compound Arithmetic op=OR(w225, w223) -> (w224:bool)
      }
      frame True {
      }
    }
    n153 = case shown="False" w219 {
      tunnel: w220 -> [w241 _]
      tunnel: [w240 w279] -> w216
      tunnel: w212 -> [w235 w279]
      tunnel: w215 -> [w231 _]
      tunnel: [w239 w278] -> w214
      tunnel: w213 -> [w233 w278]
      frame False {
        w236 = u32 12  # Max Rate (ms)
        # "Data received OR running in simulation mode"
        n154 = Increment(x=w235) -> (x+1=w234:i32)
        n155 = Tick Count (ms)() -> (millisecond timer value=w238:u32)
        n156 = Subtract(x=w238, y=w233) -> (x-y=w237:u32)
        n157 = Greater Or Equal?(x=w237, y=w236) -> (x >= y?=w232:bool)
        n158 = case shown="True" w232 {
          tunnel: w241 -> [_ w250]
          tunnel: [w243 w249] -> w240
          tunnel: [w242 w248] -> w239
          tunnel: w234 -> [w243 w247]
          tunnel: w233 -> [w242 _]
          tunnel: w231 -> [_ w246]
          frame False {
            # "Prevents the graphs from updating at over 62Hz."
          }
          frame True {
            # "Prevents the graphs from updating at over 62Hz."
            n159 = flat-sequence {
              tunnel: w247 -> [w259]
              tunnel: w250 -> [w260]
              tunnel: [w259] -> w245
              tunnel: w246 -> [w258]
              tunnel: [w258] -> w244
              tunnel: [w276] -> w249
              tunnel: w245 -> [w276]
              tunnel: [w275] -> w248
              tunnel: w244 -> [w273]
              frame #0 {
                # "Cannot be subVI'd because of an NI vision bug and limitation."
                n160 = local read "Left Channel"() -> (w262:T1)
                n161 = local read "Right Channel"() -> (w261:T1)
                n162 = call "Live window-Refresh graphs.vi"("Visible(Grid)"="Show REF Image Right", "Right Channel"=w261, "Left Channel"=w262, "Element to queue"=w260) -> ("Right image"=w256:T3, "Enable right image"=w252:bool, "Enable left image"=w254:bool, "Left image"=w257:T3)  [unwired: 4 in]
                n163 = call <userlib>:"Change Detector.vi"("Value"=w252) -> ("Changed?"=w253:bool)
                n164 = case shown="True" w253 {
                  tunnel: w252 -> [_ w264]
                  frame False {
                  }
                  frame True {
                    n165 = case shown="True" w264 {
                      tunnel: [2 0] -> w263
                      frame False {
                      }
                      frame True {
                      }
                    }
                    n166 = property on="Right Image" class="ImageControl"("DisabledEnum"=w263) -> ()  [unwired: 2 in, 2 out]
                  }
                }
                n167 = call <userlib>:"Change Detector.vi"("Value"=w254) -> ("Changed?"=w255:bool)
                n168 = case shown="True" w255 {
                  tunnel: w254 -> [_ w268]
                  frame False {
                  }
                  frame True {
                    n169 = case shown="True" w268 {
                      tunnel: [2 0] -> w267
                      frame False {
                      }
                      frame True {
                      }
                    }
                    n170 = property on="Left Image" class="ImageControl"("DisabledEnum"=w267) -> ()  [unwired: 2 in, 2 out]
                  }
                }
                n171 = case shown="True" w254 {
                  tunnel: w257 -> [_ w272]
                  frame False {
                  }
                  frame True {
                    "Left Image" <- w272
                  }
                }
                n172 = case shown="True" w252 {
                  tunnel: w256 -> [_ w271]
                  frame False {
                  }
                  frame True {
                    "Right Image" <- w271
                  }
                }
              }
              frame #1 {
                n173 = call "Calculate refresh rate.vi"("Frame size"=w273) -> ("Refresh rate (Hz)"=→"Refresh rate (Hz)":i32)  [unwired: 9 in, 1 out]
                n174 = Tick Count (ms)() -> (millisecond timer value=w275:u32)
              }
            }
          }
        }
      }
      frame True {
        # "Timed out and not in simulation mode"
        n175 = call "Calculate frame rate.vi"() -> ("Frame rate (fps)"=→"Frame rate (Hz)":dbl)  [unwired: 11 in]
      }
    }
    n176 = global read "General Globals.vi" "Stop application"() -> (w211:bool)
    n177 = local read "Stop"() -> (w210:bool)
    n178 = Compound Arithmetic op=OR(w208, w211, w210) -> (w209:bool)
    "Loop" <- w217
  }
  n179 = flat-sequence {
    tunnel: w25 -> [_]
    tunnel: w26 -> [_]
    frame #0 {
      n180 = call "fgv_Bcknd Imaging window status.vi"("Function"=Read_Write_Enum."Write", "Background MovCor window is open"=FALSE) -> ()  [unwired: 8 in, 2 out]
    }
    frame #1 {
      n181 = global write "General Globals.vi" "Stop ref imaging window"(FALSE ("Stop ref imaging window")) -> ()
      n182 = local write "Stop"(FALSE ("Stop")) -> ()
      n183 = invoke class="VI" method="FP.Close"() -> (error out=w284:errorcluster)  [unwired: 3 in, 2 out]
      n184 = call <vilib>:"Clear Errors.vi"("error in (no error)"=w284) -> ()  [unwired: 5 in, 2 out]
    }
    frame #2 {
      n185 = disable-structure shown="Disabled" {
        frame Disabled {
          n186 = Request Deallocation(TRUE ("flag")) -> ()
        }
        frame Enabled {
        }
      }
    }
  }
  n187 = call "Save_Windows_Bounds.vi"("Window Name (i.e. Key)"=w30, "Front Panel Window:Open"=FALSE, "Window VI's Ref"=w28) -> ()  [unwired: 8 in, 1 out]
